vi "Conveyer Belt Count.vi"(1 "Conveyer Belt Info":T1) -> (0 "Conveyer Belt Info Out":T1)   [LabVIEW 2012]
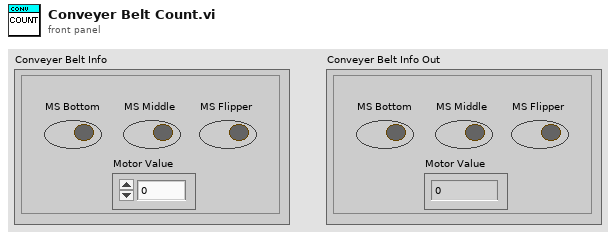
[diagram p1: front panel]
types:
  T1 = cluster{"MS Bottom":bool, "MS Middle":bool, "MS Flipper":bool, "Motor Value":dbl}
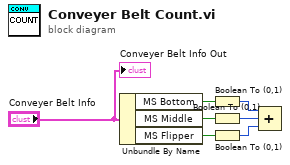
[diagram p0: block diagram]
diagram:
  n1 = Unbundle By Name("Conveyer Belt Info") -> ("MS Bottom"=w6:bool, "MS Middle"=w5:bool, "MS Flipper"=w4:bool)
  n2 = Boolean To (0,1)(Boolean=w6) -> (0, 1=w3:i16)
  n3 = Boolean To (0,1)(Boolean=w5) -> (0, 1=w2:i16)
  n4 = Boolean To (0,1)(Boolean=w4) -> (0, 1=w1:i16)
  n5 = Compound Arithmetic op=ADD(w3, w2, w1) -> ()  [unwired: 1 out]
  "Conveyer Belt Info Out" <- "Conveyer Belt Info"
